vi "Datasheet Lookup FID for Custom.vi"(1 "sxFieldId":string[](array[string]), 2 "Display Names":string[](array[string]), 3 "Modified Report Parameters":T1, 4 "Original Parameters":T1) -> (0 "Report Parameters":T1)   [LabVIEW 2011]
uses:
  ITK EXT/utils/keyedarr.llb/Keyed Array.ctl
  ITK EXT/utils/strutil.llb/Case Matching.ctl
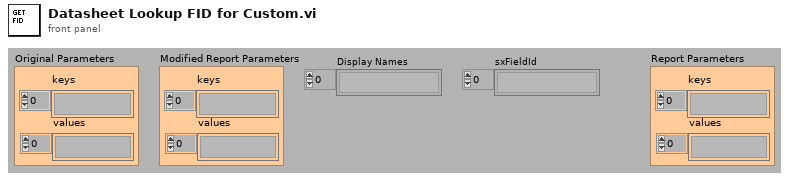
[diagram p1: front panel]
types:
  T1 = typedef "Keyed Array.ctl" = cluster{"keys":string[], "values":string[]}
  T2 = typedef "Case Matching.ctl" = enum16{"a != A", "a == A", "system"}
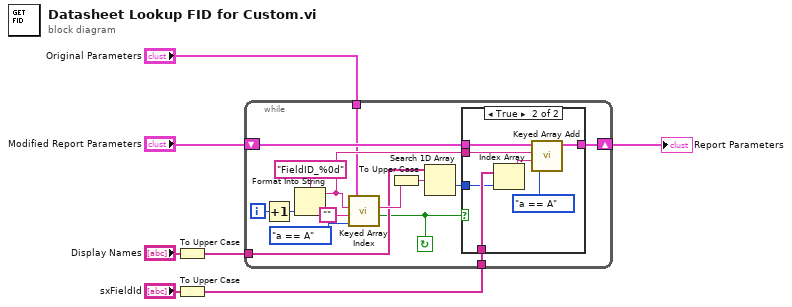
[diagram p0: block diagram]
diagram:
  n1 = To Upper Case(1:"Display Names") -> (0:w3:string[])
  n2 = To Upper Case(1:"sxFieldId") -> (0:w1:string[])
  n3 = while {
    shift-right: [w16] -> w7
    shift-left: "Modified Report Parameters" -> [w17]
    tunnel: w1 -> [w13]
    tunnel: w3 -> [w11]
    tunnel: "Original Parameters" -> [w8]
    i -> [w18]
    stop <- w9 continue-if-true
    n4 = Increment(x=w18) -> (x+1=w22:i32)
    n5 = Format Into String(format string="FieldID_%0d", w22) -> (resulting string=w15:string)  [unwired: 2 in, 1 out]
    n6 = call "Keyed Array Index.vi"("case matching (sensitive)"=Case_Matching."a == A", "default value"="", "key"=w15, "array in"=w8) -> ("valid key"=w9:bool, "value"=w14:string)  [unwired: 2 out]
    n7 = To Upper Case(1:w14) -> (0:w10:string)
    n8 = Search 1D Array(1D array=w11, element=w10) -> (index of element=w12:i32)  [unwired: 1 out]
    n9 = case shown="True" w9 {
      tunnel: w17 -> [w23 w30]
      tunnel: [w23 w29] -> w16
      tunnel: w15 -> [_ w27]
      tunnel: w13 -> [_ w26]
      tunnel: w12 -> [_ w24]
      frame False {
      }
      frame True {
        n10 = Index Array(array=w26, index=w24) -> (element=w25:string)
        n11 = call "Keyed Array Add.vi"("case matching (sensitive)"=Case_Matching."a == A", "value"=w25, "key"=w27, "array in"=w30) -> ("array out"=w29:T1)  [unwired: 3 out]
      }
    }
  }
  "Report Parameters" <- w7
